vi "111-Login.vi"() -> ()   [LabVIEW 2019]
uses:
  <vilib>/Utility/error.llb/DialogType.ctl
  <vilib>/addons/database/Connection.llb/DB Tools Open Connec (String).vi
  <vilib>/addons/database/Connection.llb/Conn Execute.vi
  <vilib>/addons/database/Recordset.llb/Rec Fetch Recordset Data (R).vi
  <vilib>/addons/database/Recordset.llb/Rec Destroy - Connection.vi
  <vilib>/addons/database/NI_Database_API.lvlib
panel:
  in  "登陆":bool
  in  "密   码":string
  out "数据库连接成功":bool
  in  "联机模式":enum16{"单机版", "网络版"}(ring)
  in  "用户名":string
  # "数据库状态"
  # "调阀台"
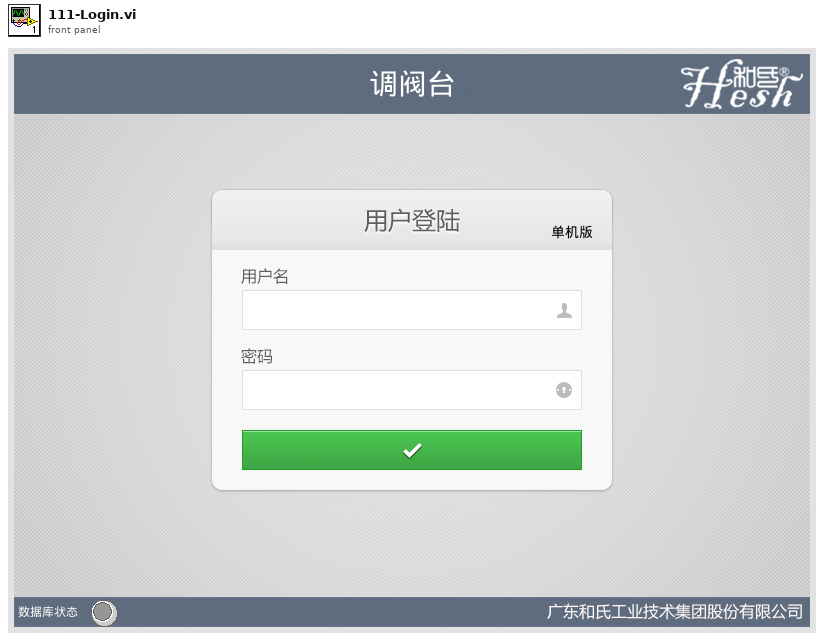
[diagram p1: front panel]
types:
  T1 = enum32{"Invalid", "Standard", "Closed", "Hidden", "Minimized", "Maximized"}
  T2 = typedef "DialogType.ctl" = u16
  T3 = typedef "eventvkey.ctl" = enum16{"ASCII", "Enter", "Return", "Shift", "Ctrl", "Alt", "Cmd", "Opt", "Caps", "NumLock", "Clear", "Break", "Up", "Down", "Left", "Right", "Insert", "Delete", "Home", "End", "PageUp", "PageDown", "Escape", "Help", "Pause", "ScrollLock", "F1", "F2", "F3", "F4", "F5", "F6", "F7", "F8", "F9", "F10", "F11", "F12", "F13", "F14", "F15", "F16", "F17", "F18", "F19", "F20", "F21", "F22", "F23", "F24", "Play", "VolumeUp", "VolumeDown", "Mute", "Two Byte Char"}
  T4 = typedef "NI_Database_API.lvlib/Conn ObjectReference.ctl" = refnum<k1>
  T5 = typedef "NI_Database_API.lvlib/Rec ObjectReference.ctl" = refnum<k1>
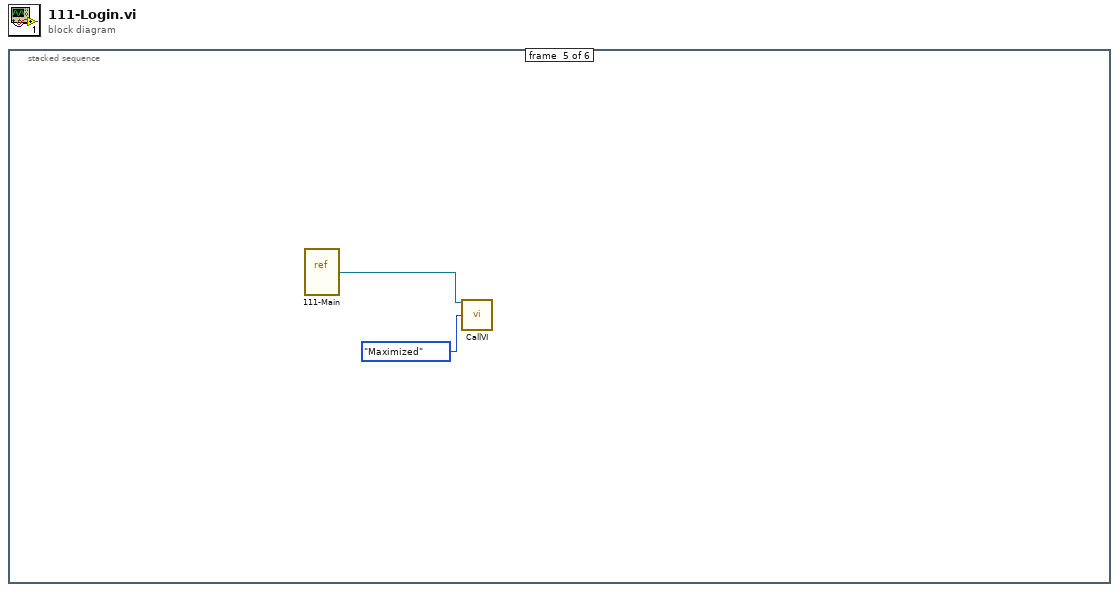
[diagram p0: block diagram]
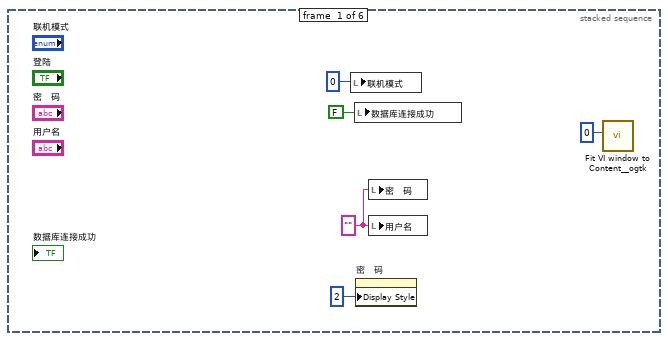
[diagram p2: hidden frame]
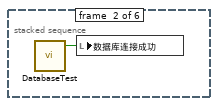
[diagram p3: hidden frame]
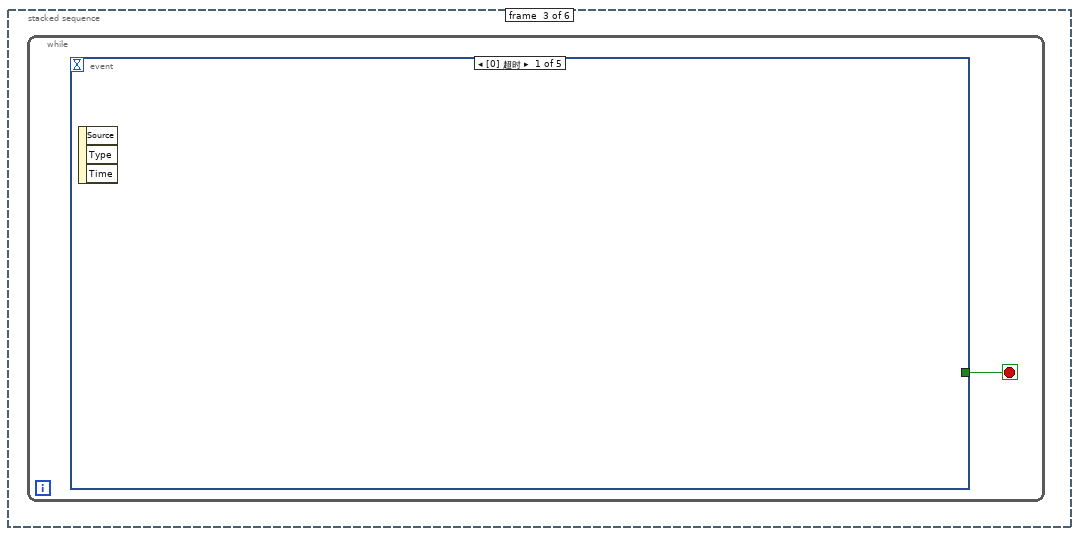
[diagram p4: hidden frame]
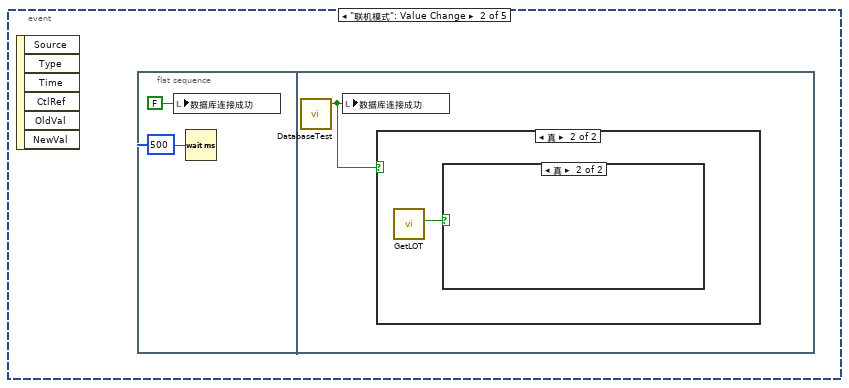
[diagram p5: hidden frame]
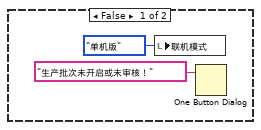
[diagram p7: hidden frame]
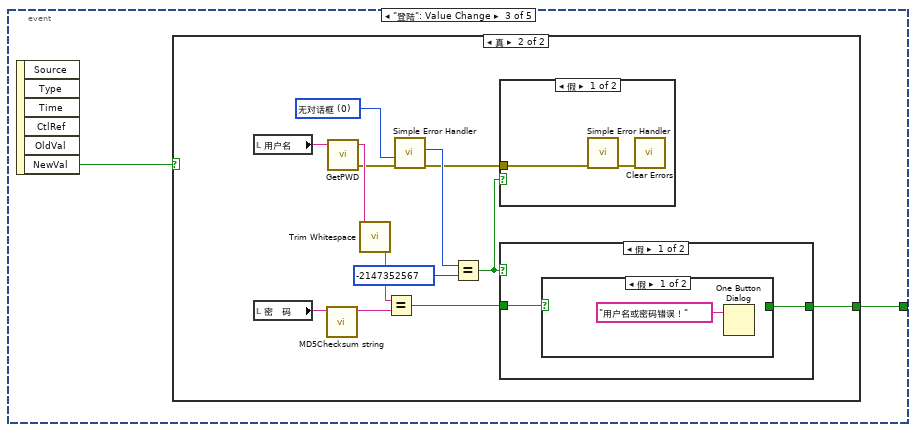
[diagram p8: hidden frame]
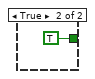
[diagram p10: hidden frame]
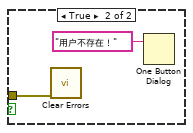
[diagram p12: hidden frame]
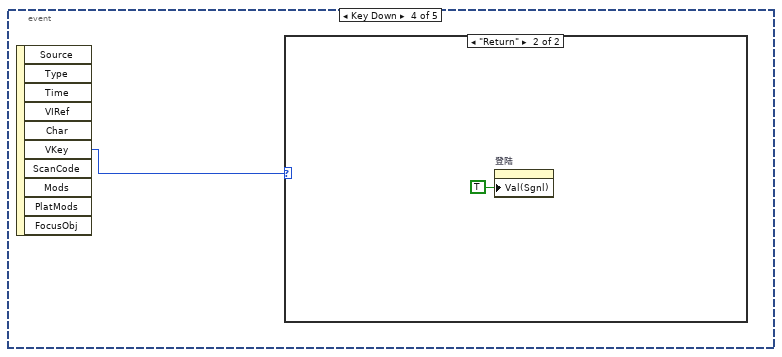
[diagram p13: hidden frame]
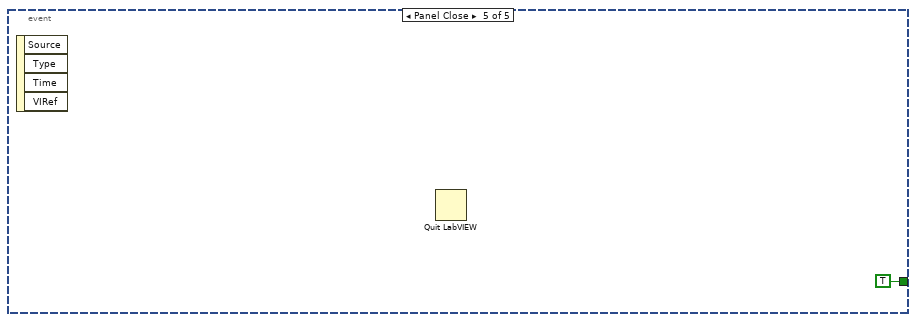
[diagram p15: hidden frame]
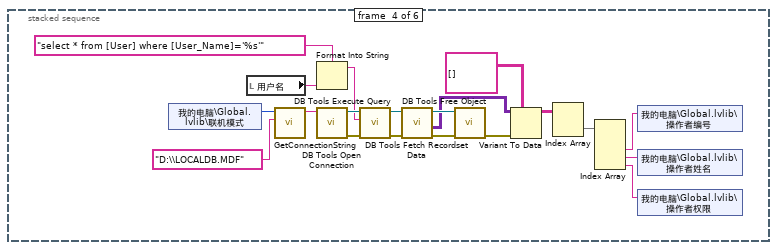
[diagram p16: hidden frame]
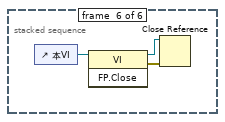
[diagram p17: hidden frame]
diagram:
  n1 = stacked-sequence {
    frame #0 {
      w3 = ""
      n2 = local write "联机模式"(u16 0 ("程序版本")) -> ()
      n3 = local write "数据库连接成功"(FALSE ("数据库连接成功")) -> ()
      n4 = property on="密   码" class="Str"("Display Style"=u32 2 ("显示样式")) -> ()  [unwired: 2 in, 2 out]
      n5 = local write "密   码"(w3) -> ()
      n6 = local write "用户名"(w3) -> ()
      n7 = call <userlib>:"Fit VI window to Content__ogtk.vi"("border spacing (2 px)"=0) -> ()  [unwired: 5 in, 2 out]
    }
    frame #1 {
      n8 = call "DatabaseTest.vi"() -> ("数据库连接成功"=w6:bool)  [unwired: 4 in, 1 out]
      n9 = local write "数据库连接成功"(w6) -> ()
    }
    frame #2 {
      n10 = while {
        stop <- w7 stop-if-true
        n11 = event shown="[0] 超时" {
          selector: _ -> [_ _ _ _ _]
          dyn-events: _ -> [_ _ _ _ _]
          timeout: _ -> [_ _ _ _ _]
          tunnel: [_ _ w14 _ TRUE] -> w7
          event Timeout {
            n12 = event-data() -> ()  [unwired: 1 in, 3 out]
          }
          event "联机模式": Value Change {
            n13 = event-data() -> ()  [unwired: 1 in, 6 out]
            n14 = flat-sequence {
              frame #0 {
                n15 = local write "数据库连接成功"(FALSE ("数据库连接成功")) -> ()
                n16 = Wait (ms)(milliseconds to wait=u32 500 ("等待时间（毫秒）")) -> ()  [unwired: 1 out]
              }
              frame #1 {
                n17 = call "DatabaseTest.vi"() -> ("数据库连接成功"=w10:bool)  [unwired: 4 in, 1 out]
                n18 = local write "数据库连接成功"(w10) -> ()
                n19 = case shown="真" w10 {
                  frame False {
                  }
                  frame True {
                    n20 = call "GetLOT.vi"() -> ("生产批次有效"=w11:bool)  [unwired: 9 in, 2 out]
                    n21 = case shown="真" w11 {
                      frame False {
                        n22 = local write "联机模式"(enum16{"单机版", "网络版"}."单机版" ("联机模式")) -> ()
                        n23 = One Button Dialog(message="生产批次未开启或未审核！" ("消息")) -> ()  [unwired: 1 in, 1 out]
                      }
                      frame True {
                      }
                    }
                  }
                }
              }
            }
          }
          event "登陆": Value Change {
            n24 = event-data() -> ("NewVal"=w15:bool)  [unwired: 1 in, 5 out]
            n25 = case shown="真" w15 {
              tunnel: [_ w19] -> w14
              frame False {
              }
              frame True {
                w24 = T2 0 items=["无对话框", "确定信息", "继续或停止信息", "确定信息＋警告", "继续/停止+警告"] ("type of dialog (OK msg:1)")
                n26 = local read "用户名"() -> (w26:string)
                n27 = local read "密   码"() -> (w17:string)
                n28 = call <vilib>:"MD5Checksum string.vi"("Message String"=w17) -> ("MD5 message-digest"=w18:string)  [unwired: 10 in]
                n29 = call "GetPWD.vi"("User_Name"=w26) -> ("error out"=w25:errorcluster, "Password"=w28:string)  [unwired: 2 in, 1 out]
                n30 = call <vilib>:"Trim Whitespace.vi"("string"=w28) -> ("trimmed string"=w16:string)  [unwired: 1 in]
                n31 = Equal?(x=w16, y=w18) -> (x = y?=w27:bool)
                n32 = call <vilib>:"Simple Error Handler.vi"("type of dialog (OK msg:1)"=w24, "error in (no error)"=w25) -> ("code out"=w23:i32, "error out"=w21:errorcluster)  [unwired: 3 in, 3 out]
                n33 = Equal?(x=w23, y=-2147352567) -> (x = y?=w20:bool)
                n34 = case shown="假" w20 {
                  tunnel: w21 -> [w34 w35]
                  frame False {
                    n35 = call <vilib>:"Simple Error Handler.vi"("error in (no error)"=w34) -> ("error out"=w33:errorcluster)  [unwired: 4 in, 4 out]
                    n36 = call <vilib>:"Clear Errors.vi"("error in (no error)"=w33) -> ()  [unwired: 5 in, 2 out]
                  }
                  frame True {
                    n37 = call <vilib>:"Clear Errors.vi"("error in (no error)"=w35) -> ()  [unwired: 5 in, 2 out]
                    n38 = One Button Dialog(message="用户不存在！" ("消息")) -> ()  [unwired: 1 in, 1 out]
                  }
                }
                n39 = case shown="假" w20 {
                  tunnel: w27 -> [w30 _]
                  tunnel: [w29 _] -> w19
                  frame False {
                    n40 = case shown="假" w30 {
                      tunnel: [_ TRUE] -> w29
                      frame False {
                        n41 = One Button Dialog(message="用户名或密码错误！" ("消息")) -> ()  [unwired: 1 in, 1 out]
                      }
                      frame True {
                      }
                    }
                  }
                  frame True {
                  }
                }
              }
            }
          }
          event Key Down {
            n42 = event-data() -> ("VKey"=w37:T3)  [unwired: 1 in, 9 out]
            n43 = case shown="\"Return\"" w37 {
              frame "ASCII", Default {
              }
              frame "Return" {
                n44 = property on="登陆" class="Bool (严格)"("Val(Sgnl)"=TRUE ("值(信号)")) -> ()  [unwired: 2 in, 2 out]
              }
            }
          }
          event Panel Close {
            n45 = event-data() -> ()  [unwired: 1 in, 4 out]
            n46 = Quit LabVIEW() -> ()  [unwired: 1 in]
          }
        }
      }
    }
    frame #3 {
      n47 = shared-variable "我的电脑\\Global.lvlib\\联机模式"() -> (w40:i16)  [unwired: 1 in, 1 out]
      n48 = local read "用户名"() -> (w42:string)
      n49 = call "GetConnectionString.vi"("Database Name"="D:\\LOCALDB.MDF", "连接模式"=w40) -> ("连接字符串"=w58:string)  [unwired: 4 in, 1 out]
      n50 = Format Into String(format string="select * from [User] where [User_Name]='%s'", w42) -> (resulting string=w41:string)  [unwired: 2 in, 1 out]
      n51 = call-poly <vilib>:"DB Tools Open Connection.vi"("connection information"=w58) -> ("error out"=w57:errorcluster, "connection reference"=w56:T4)  [unwired: 7 in]
      n52 = call-poly <vilib>:"DB Tools Execute Query.vi"("error in (no error)"=w57, "SQL query"=w41, "connection reference"=w56) -> ("error out"=w53:errorcluster, "recordset reference"=w55:T5)  [unwired: 5 in]
      n53 = call-poly <vilib>:"DB Tools Fetch Recordset Data.vi"("error in (no error)"=w53, "recordset reference"=w55) -> ("error out"=w52:errorcluster, "recordset data"=w50:variant[][], "recordset reference out"=w54:T5)  [unwired: 3 in]
      n54 = call-poly <vilib>:"DB Tools Free Object.vi"("error in (no error)"=w52, "recordset reference"=w54) -> ("error out"=w51:errorcluster)  [unwired: 8 in, 1 out]
      n55 = Variant To Data(error in=w51, type=string[][] [], Variant=w50) -> (data=w48:string[][])  [unwired: 1 out]
      n56 = Index Array(array=w48) -> (element=w47:string[])  [unwired: 2 in]
      n57 = Index Array(array=w47) -> (element #2=w44:string, element #3=w45:string, element #4=w46:string)  [unwired: 4 in, 1 out]
      n58 = shared-variable "我的电脑\\Global.lvlib\\操作者编号"(w44) -> ()  [unwired: 1 in, 1 out]
      n59 = shared-variable "我的电脑\\Global.lvlib\\操作者姓名"(w45) -> ()  [unwired: 1 in, 1 out]
      n60 = shared-variable "我的电脑\\Global.lvlib\\操作者权限"(w46) -> ()  [unwired: 1 in, 1 out]
    }
    frame #4 {
      n61 = vi-ref "111-Main.vi"() -> (w60:refnum<vi>)
      n62 = call "CallVI.vi"("VI引用"=w60, "状态"=T1."Maximized") -> ()  [unwired: 11 in, 3 out]
    }
    frame #5 {
      n63 = control-ref of="本VI"() -> (w62:refnum<vi>)
      n64 = invoke class="VI" method="FP.Close"(reference=w62) -> (reference out=w63:refnum<vi>, error out=w64:errorcluster)  [unwired: 2 in, 1 out]
      n65 = Close Reference(reference=w63, error in (no error)=w64) -> ()  [unwired: 1 out]
    }
  }
